vi "ReadConfig.vi"() -> ()   [LabVIEW 2020]
uses:
  <vilib>/Utility/config.llb/Read Key (Boolean).vi
  <vilib>/Utility/config.llb/Read Key (Double).vi
  <vilib>/Utility/config.llb/Read Key (Path).vi
  <vilib>/Utility/config.llb/Read Key (String).vi
  <vilib>/Utility/config.llb/NI_LVConfig.lvlib
panel:
  out "Path Value":path
  out "Numeric":dbl format="%0.2f"
  out "Boolean":bool
  out "String 2":string
  out "String 1":string
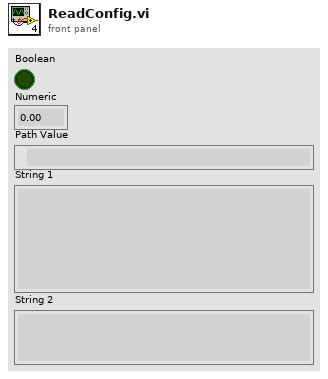
[diagram p1: front panel]
types:
  T1 = typedef "NI_LVConfig.lvlib/Config Data RefNum.ctl" = refnum<k1>
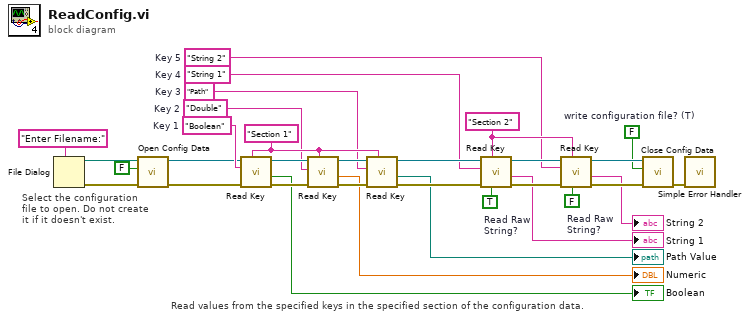
[diagram p0: block diagram]
diagram:
  w2 = FALSE  # write configuration file? (T)
  w4 = TRUE  # Read Raw String?
  w6 = FALSE  # Read Raw String?
  w15 = "String 2"  # Key 5
  w16 = "String 1"  # Key 4
  w17 = "Path"  # Key 3
  w18 = "Double"  # Key 2
  w19 = "Boolean"  # Key 1
  w20 = "Section 2" ("section")
  w21 = "Section 1" ("section")
  # "Read values from the specified keys in the specified section of the configuration data."
  # "Select the configuration file to open. Do not create it if it doesn't exist."
  n1 = File Dialog(7:"Enter Filename:" ("Prompt")) -> (0:w1:errorcluster, 3:w22:path)  [unwired: 1 in, 7 out]
  n2 = call <vilib>:"Open Config Data.vi"("error in (no error)"=w1, "create file if necessary (T)"=FALSE ("create file if necessary? (T)"), "configuration file path"=w22) -> ("error out"=w13:errorcluster, "refnum"=w12:T1)  [unwired: 6 in, 1 out]
  n3 = call-poly <vilib>:"Read Key.vi"("section"=w21, "error in (no error)"=w13, "key"=w19, "refnum"=w12) -> ("error out"=w32:errorcluster, "value"=→"Boolean":bool, "refnum out"=w30:T1)  [unwired: 1 in, 4 out]
  n4 = call-poly <vilib>:"Read Key.vi"("section"=w21, "error in (no error)"=w32, "key"=w18, "refnum"=w30) -> ("error out"=w27:errorcluster, "value"=→"Numeric":dbl, "refnum out"=w28:T1)  [unwired: 1 in, 4 out]
  n5 = call-poly <vilib>:"Read Key.vi"("section"=w21, "error in (no error)"=w27, "key"=w17, "refnum"=w28) -> ("error out"=w31:errorcluster, "value"=→"Path Value":path, "refnum out"=w29:T1)  [unwired: 1 in, 4 out]
  n6 = call-poly <vilib>:"Read Key.vi"("read raw string? (F)"=w4, "section"=w20, "error in (no error)"=w31, "key"=w16, "refnum"=w29) -> ("error out"=w24:errorcluster, "value"=→"String 1":string, "refnum out"=w23:T1)  [unwired: 1 in, 3 out]
  n7 = call-poly <vilib>:"Read Key.vi"("read raw string? (F)"=w6, "section"=w20, "error in (no error)"=w24, "key"=w15, "refnum"=w23) -> ("error out"=w26:errorcluster, "value"=→"String 2":string, "refnum out"=w25:T1)  [unwired: 1 in, 3 out]
  n8 = call <vilib>:"Close Config Data.vi"("error in (no error)"=w26, "write file if changed (T)"=w2, "refnum"=w25) -> ("error out"=w14:errorcluster)  [unwired: 8 out]
  n9 = call <vilib>:"Simple Error Handler.vi"("error in (no error)"=w14) -> ()  [unwired: 1 in, 8 out]
